vi "Reconnect.vi"(0 "STOMP in":refnum<class "STOMP.lvclass">, 4 "timeout ms (10000)":i32=20000, 5 "error in (no error)":errorcluster) -> (14 "STOMP out":refnum<class "STOMP.lvclass">, 19 "error out":errorcluster)   [LabVIEW 2017, in "STOMP.lvclass"]
uses:
  STOMP.lvclass
  STOMP.lvclass/STOMP.ctl
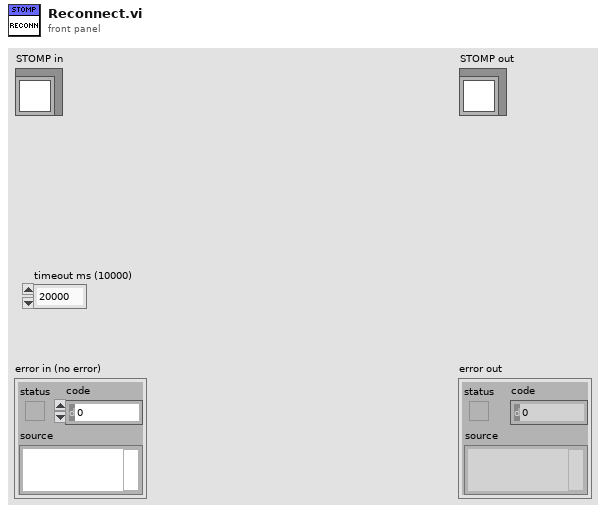
[diagram p1: front panel]
types:
  T1 = typedef "LabVIEW STOMP.lvlib/STOMP.lvclass/ObjectAttributes.ctl" = cluster{"address":string, "port":u16, "ConnectionRef":refnum<k5>, "messageQueue":refnum<queue>, "receiptQueue":refnum<queue>, "errorQueue":refnum<queue>, "sendQueue":refnum<queue>, "currentReceiptNumber":u64, "currentSubscriptionId":u64, "closeConnection":bool, "activeSubscriptions":T2[]}
  T2 = typedef "Type_ActiveSubscription.ctl" = cluster{"id":u64, "receipt":bool, "Destination":string, "ack":T3, "headers":T4[]}
  T3 = typedef "Type_AckHeader.ctl" = enum16{"auto", "client", "client-individual"}
  T4 = typedef "LabVIEW STOMP.lvlib/STOMP.lvclass/Type_FrameHeader.ctl" = cluster{"Header":string, "Value":string}
  T5 = typedef "STOMP.lvclass/Type_ServerFrame.ctl" = cluster{"Type":T6, "Headers":cluster{"Header":string, "Value":string}[], "Body":string}
  T6 = typedef "STOMP.lvclass/Type_ServerFrameType.ctl" = enum16{"Undefined", "MESSAGE", "CONNECTED", "RECEIPT", "ERROR"}
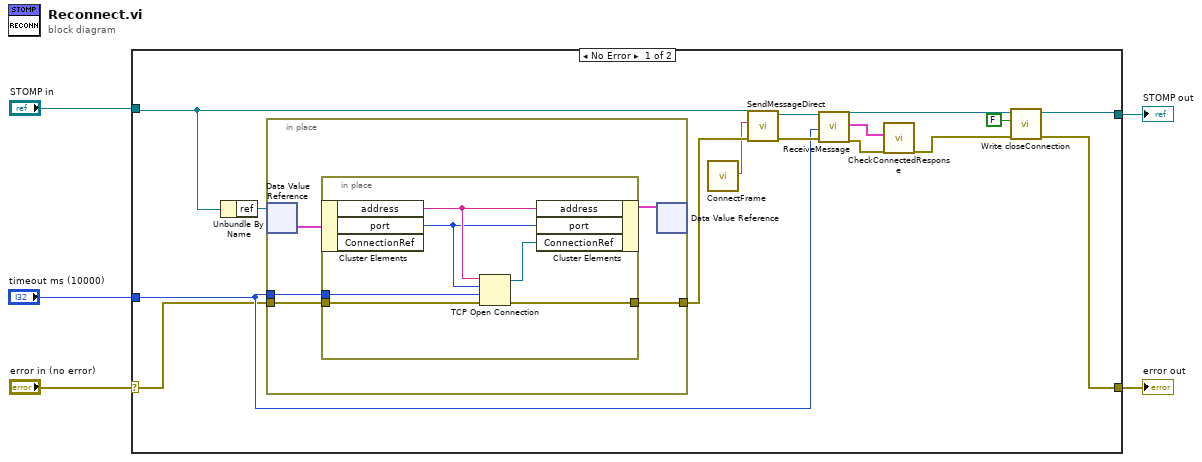
[diagram p0: block diagram]
diagram:
  n1 = case shown="No Error" "error in (no error)" {
    selector: "error in (no error)" -> [w11 w33]
    tunnel: [w8 w33] -> w4
    tunnel: [w7 w32] -> w2
    tunnel: "STOMP in" -> [w13 w32]
    tunnel: "timeout ms (10000)" -> [w14 _]
    frame No Error {
      n2 = Unbundle By Name(w13) -> ("ref"=w12:refnum<data-value>)
      n3 = in-place {
        in-place-border: [w25] -> w20
        in-place-border: w14 -> [w24]
        in-place-border: w11 -> [w21]
        n4 = in-place-dvr #1(w12) -> (w23:T1)  [unwired: 1 out]
        n5 = in-place {
          in-place-border: w24 -> [w29]
          in-place-border: [w27] -> w25
          in-place-border: w21 -> [w26]
          n6 = in-place-cluster #2(w23) -> ("address"=w31:string, "port"=w30:u16)  [unwired: 1 out]
          n7 = TCP Open Connection(address=w31, remote port or service name=w30, timeout ms (60000)=w29, error in (no error)=w26) -> (connection ID=w28:refnum<k5>, error out=w27:errorcluster)  [unwired: 1 in]
          n8 = in-place-cluster #2("address"=w31, "port"=w30, "ConnectionRef"=w28) -> (w22:T1)
        }
        n9 = in-place-dvr #1(w22) -> ()  [unwired: 2 out]
      }
      n10 = call "ConnectFrame.vi"() -> ("Connect Frame"=w19:string)  [unwired: 19 in]
      n11 = call-dynamic "SendMessageDirect.vi"("error in (no error)"=w20, "data in"=w19, "STOMP in"=w13) -> ("error out"=w17:errorcluster, "STOMP out"=w18:refnum<class "STOMP.lvclass">)  [unwired: 7 in]
      n12 = call-dynamic "ReceiveMessage.vi"("STOMP in"=w18, "timeout ms (25000)"=w14, "error in (no error)"=w17) -> ("STOMP out"=w10:refnum<class "STOMP.lvclass">, "ServerFrame"=w16:T5, "error out"=w15:errorcluster)  [unwired: 14 in]
      n13 = call "CheckConnectedResponse.vi"("message"=w16, "error in (no error)"=w15) -> ("error out"=w9:errorcluster)  [unwired: 17 in]
      n14 = call-dynamic "Write closeConnection.vi"("error in (no error)"=w9, "closeConnection"=FALSE, "STOMP in"=w10) -> ("error out"=w8:errorcluster, "STOMP out"=w7:refnum<class "STOMP.lvclass">)  [unwired: 7 in]
    }
    frame Error {
    }
  }
  "error out" <- w4
  "STOMP out" <- w2
